vi "PD.vi"(7 "dt (s)":dbl=0.05 format="%#_13g", 10 "ENC":i32[](array[numeric]), 11 "SET":dbl[](array[numeric])) -> (3 "output":dbl[](array[numeric]))   [LabVIEW 2017]
uses:
  <vilib>/addons/control/pid/pid.llb/PID (DBL Array).vi
  <vilib>/addons/control/pid/NI_PID_pid.lvlib
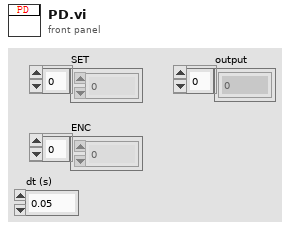
[diagram p1: front panel]
types:
  T1 = cluster{"proportional gain (Kc)":dbl, "integral time (Ti, min)":dbl, "derivative time (Td, min)":dbl}
  T2 = cluster{"proportional gain (Kc)":dbl, "integral time (Ti, min)":dbl, "derivative time (Td, min)":dbl}[]
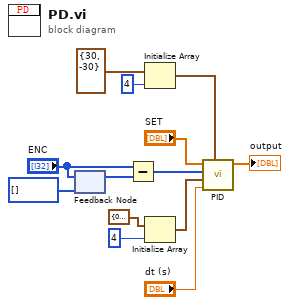
[diagram p0: block diagram]
diagram:
  n1 = feedback-in #1("ENC") -> ()
  n2 = feedback #1(i32[] [] ("ENC")) -> (w2:i32[])
  n3 = Subtract(x="ENC", y=w2) -> (x-y=w4:i32[])
  n4 = Initialize Array(cluster{"output high":i32, "output low":i32} {"output high"=30, "output low"=-30} ("output range"), 4 ("维数大小")) -> (w12:cluster{"output high":i32, "output low":i32}[])
  n5 = Initialize Array(T1 {"proportional gain (Kc)"=0.0009999999999999966, "integral time (Ti, min)"=0.0, "derivative time (Td, min)"=0.06399999999999995} ("PID gains 2"), 4 ("维数大小")) -> (w8:T2)
  n6 = call-poly <vilib>:"PID.vi"("output range"=w12, "dt (s)"="dt (s)", "PID gains"=w8, "process variable"=w4, "setpoint"="SET") -> ("output"=→"output":dbl[])  [unwired: 5 in, 1 out]
